vi "Lixo2.vi"() -> ()   [LabVIEW 2018]
panel:
  in  "Numeric":u16 format="%x"
  out "sum":i16
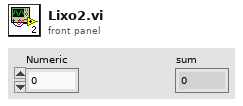
[diagram p1: front panel]
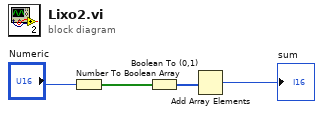
[diagram p0: block diagram]
diagram:
  n1 = Number To Boolean Array(number="Numeric") -> (Boolean array=w1:bool[])
  n2 = Boolean To (0,1)(Boolean=w1) -> (0, 1=w4:i16[])
  n3 = Add Array Elements(numeric array=w4) -> (sum=→"sum":i16)
